vi "Init I2C Resources.vi"(8 "error in (no error)":errorcluster, 11 "Session in":refnum<class "Session.lvclass">) -> (0 "error out":errorcluster, 3 "Session out":refnum<class "Session.lvclass">)   [LabVIEW 2024, in "CTI.lvlib" / "Session.lvclass"]
uses:
  Session.lvclass
  I2C Number.ctl
  I2C/I2C.lvclass
  Session.lvclass/Session.ctl
  CTI.lvlib
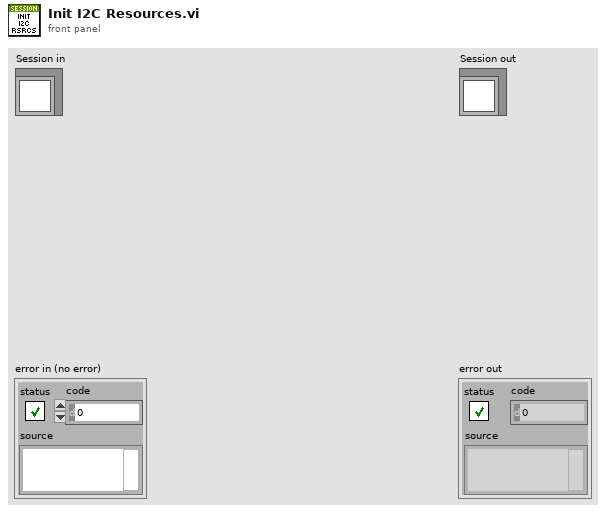
[diagram p1: front panel]
types:
  T1 = typedef "CTI.lvlib/I2C Number.ctl" = i8
  T2 = typedef "CTI.lvlib/Available I2C.ctl" = cluster{"I2C #":T1, "SCL GPIOs":T3[], "SDA GPIOs":T3[]}
  T3 = typedef "CTI.lvlib/GPIO Number.ctl" = i8
  T4 = typedef "CTI.lvlib/Session.lvclass/Resources.ctl" = cluster{"GPIO":map{T3, refnum<class "GPIO.lvclass">}, "AI":map{T5, refnum<class "AI.lvclass">}, "PWM":map{T3, refnum<class "PWM.lvclass">}, "UART":map{T6, refnum<class "UART.lvclass">}, "I2C":map{T1, refnum<class "I2C.lvclass">}, "SPI":map{T7, refnum<class "SPI.lvclass">}, "SPI CS":map{T3, refnum<class "SPI CS.lvclass">}}
  T5 = typedef "CTI.lvlib/ADC Number.ctl" = i8
  T6 = typedef "CTI.lvlib/UART Number.ctl" = i8
  T7 = typedef "CTI.lvlib/SPI Number.ctl" = i8
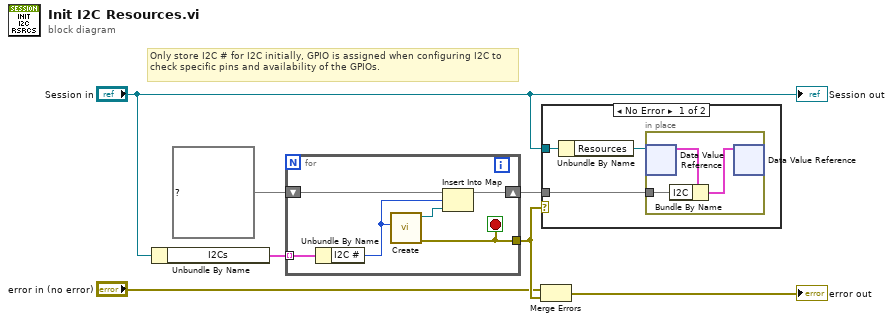
[diagram p0: block diagram]
diagram:
  # "Only store I2C # for I2C initially, GPIO is assigned when configuring I2C to check specific pins and availability of the GPIOs."
  n1 = Unbundle By Name("Session in") -> ("I2Cs"=w3:T2[])
  n2 = for {
    tunnel: w3 -> [w10] mode=indexing
    shift-right: [w12] -> w4
    shift-left: map{T1, refnum<class "I2C.lvclass">} {} ("I2C") -> [w13]
    tunnel: [w11] -> w7
    stop <- w11 stop-if-true
    n3 = Unbundle By Name(w10) -> ("I2C #"=w8:T1)
    n4 = call "Create.vi"("I2C #"=w8) -> ("error out"=w11:errorcluster, "I2C out"=w9:refnum<class "I2C.lvclass">)  [unwired: 9 in]
    n5 = Insert Into Map(map in=w13, key=w8, value=w9) -> (map out=w12:map{T1, refnum<class "I2C.lvclass">})  [unwired: 2 out]
  }
  n6 = Merge Errors("error in (no error)", w7) -> (→"error out":errorcluster)
  n7 = case shown="No Error" w7 {
    tunnel: w4 -> [w14 _]
    tunnel: "Session in" -> [w16 _]
    frame No Error {
      n8 = Unbundle By Name(w16) -> ("Resources"=w15:refnum<data-value>)
      n9 = in-place {
        in-place-border: w14 -> [w17]
        n10 = in-place-dvr #1(w15) -> (w19:T4)  [unwired: 1 out]
        n11 = Bundle By Name(cluster=w19, "I2C"=w17) -> (w18:T4)
        n12 = in-place-dvr #1(w18) -> ()  [unwired: 2 out]
      }
    }
    frame Error {
    }
  }
  "Session out" <- "Session in"
